vi "Main.vi"() -> ()   [LabVIEW 2017]
doc: "The myRIO Project template acquires acceleration data from the onboard accelerometer and displays the changes of acceleration values in a waveform chart."
uses:
  Encoder Control.ctl
  <vilib>/addons/control/pid/pid.llb/PID (DBL).vi
  <vilib>/addons/control/pid/NI_PID_pid.lvlib
panel:
  in  "PID Position":T1=enum."2000"
  out "Numeric Control":i32
  out "Waveform Chart":T2(graph)
  in  "PID gains":T3={"proportional gain (Kc)"=1.0, "integral time (Ti, min)"=0.01, "derivative time (Td, min)"=0.0}
  in  "Stop Button":bool
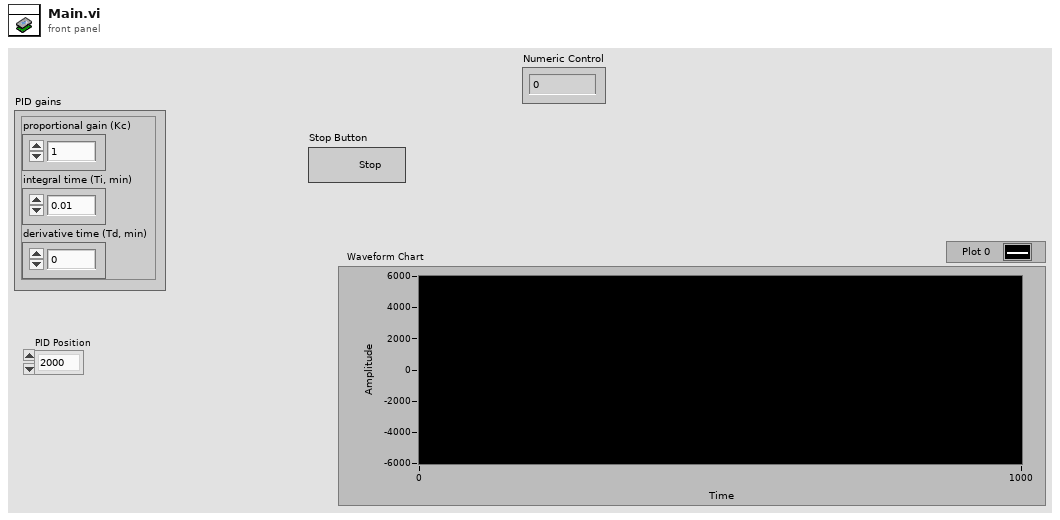
[diagram p1: front panel]
types:
  T1 = typedef "Encoder Control.ctl" = enum16{"0", "2000", "4000", "6000"}
  T2 = cluster{"Counter Value":i32, "Counter Value":i32}
  T3 = cluster{"proportional gain (Kc)":dbl, "integral time (Ti, min)":dbl, "derivative time (Td, min)":dbl}
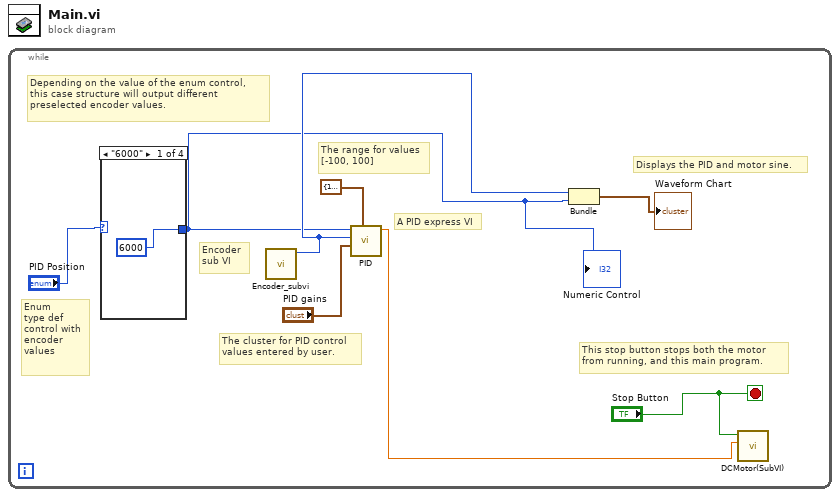
[diagram p0: block diagram]
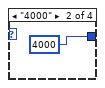
[diagram p2: hidden frame]
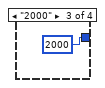
[diagram p3: hidden frame]
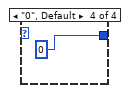
[diagram p4: hidden frame]
diagram:
  n1 = while {
    stop <- "Stop Button" stop-if-true
    # "Enum \ntype def\ncontrol with\nencoder\nvalues"
    # "This stop button stops both the motor \nfrom running, and this main program."
    # "Displays the PID and motor sine."
    # "Encoder \nsub VI"
    # "A PID express VI"
    # "The range for values\n[-100, 100]"
    # "The cluster for PID control\nvalues entered by user."
    # "Depending on the value of the enum control,\nthis case structure will output different \npreselected encoder values."
    n2 = case shown="\"6000\"" "PID Position" {
      tunnel: [6000 4000 2000 0] -> w2
      frame "6000" {
      }
      frame "4000" {
      }
      frame "2000" {
      }
      frame "0", Default {
      }
    }
    "Numeric Control" <- w2
    n3 = call "Encoder_subvi.vi"() -> ("Counter Value"=w5:i32)  [unwired: 10 in, 1 out]
    n4 = call-poly <vilib>:"PID.vi"("output range"=cluster{"output high":dbl, "output low":dbl} {"output high"=100.0, "output low"=-100.0}, "PID gains"="PID gains", "process variable"=w5, "setpoint"=w2) -> ("output"=w3:dbl)  [unwired: 6 in, 1 out]
    n5 = Bundle("Counter Value"=w5, w2) -> (→"Waveform Chart":cluster{"Counter Value":i32, i32})  [unwired: 1 in]
    n6 = call "DCMotor(SubVI).vi"("Duty Cycle (-100 to +100)"=w3, "Stop VI"="Stop Button") -> ()  [unwired: 10 in]
  }
